vi "BinanceAPI_averagePrice.vi"(0 "BinanceAPI in":refnum<class "BinanceAPI_.lvclass">, 1 "The name of the currency pair":string, 11 "error in (no error)":errorcluster) -> (4 "BinanceAPI out":refnum<class "BinanceAPI_.lvclass">, 14 "FastAveragePrice":ext, 15 "error out":errorcluster)   [LabVIEW 2022 SP3, in "BinanceAPI_.lvclass"]
doc: "Show only 5 min average price of pair of symbols."
uses:
  src/BinanceAPI_.lvclass
  src/BinanceAPI_.lvclass/BinanceAPI_.ctl
  <vilib>/regexp/Match Regular Expression.xnode
  <vilib>/httpClient/LabVIEWHTTPClient.lvlib
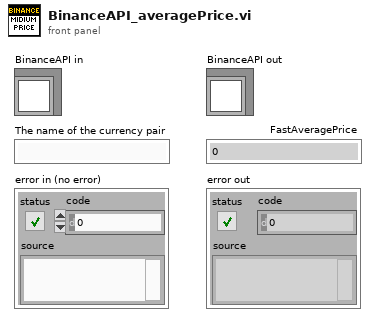
[diagram p1: front panel]
types:
  T1 = typedef "LabVIEWHTTPClient.lvlib/ClientHandle.ctl" = refnum<k1>
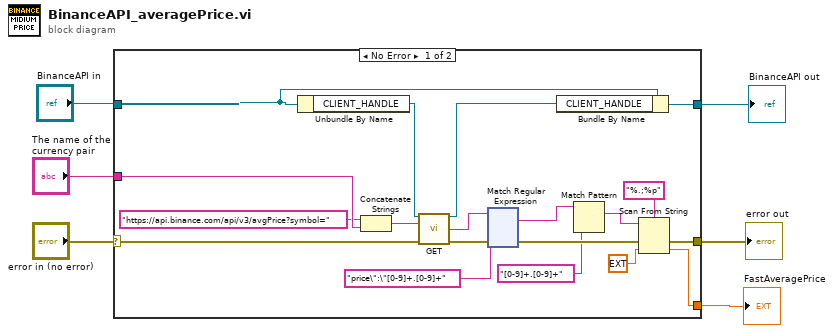
[diagram p0: block diagram]
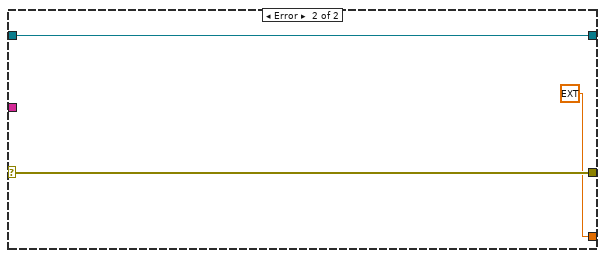
[diagram p2: hidden frame]
diagram:
  n1 = case shown="No Error" "error in (no error)" {
    selector: "error in (no error)" -> [w11 w145]
    tunnel: [w25 w145] -> w6
    tunnel: [w23 ext 0.0 ("default value 1")] -> w5
    tunnel: "The name of the currency pair" -> [w14 _]
    tunnel: "BinanceAPI in" -> [w9 w143]
    tunnel: [w8 w143] -> w1
    frame No Error {
      n2 = Unbundle By Name(w9) -> ("CLIENT_HANDLE"=w10:T1)
      n3 = Concatenate Strings("https://api.binance.com/api/v3/avgPrice?symbol=", w14) -> (w12:string)
      n4 = call <vilib>:"GET.vi"("client handle"=w10, "url"=w12, "error in (no error)"=w11) -> ("client handle out"=w7:T1, "body"=w16:string, "error out"=w17:errorcluster)  [unwired: 9 in, 1 out]
      n5 = xnode "Match Regular Expression"("input string"=w16, "regular expression"="price\":\"[0-9]+.[0-9]+", "error in"=w17) -> ("whole match"=w19:string, "error out"=w24:errorcluster)  [unwired: 3 in, 3 out]
      n6 = Bundle By Name(cluster=w9, "CLIENT_HANDLE"=w7) -> (w8:refnum<class "BinanceAPI_.lvclass">)
      n7 = Match Pattern(string=w19, regular expression="[0-9]+.[0-9]+") -> (match substring=w20:string)  [unwired: 1 in, 3 out]
      n8 = Scan From String(format string="%.;%p", input string=w20, error in=w24, default 1=ext 0.0 ("default value 1")) -> (error out=w25:errorcluster, output 1=w23:ext)  [unwired: 1 in, 2 out]
    }
    frame Error {
    }
  }
  "error out" <- w6
  "FastAveragePrice" <- w5
  "BinanceAPI out" <- w1
